vi "Enable_AFR_EGT_Graph (SubVI).vi"(0 "Leistungsgraph":refnum<vi>, 1 "AFR EGT":bool, 2 "Y-Koord. Graph-Reset-Button (782)":i32, 3 "Lambda":refnum<vi>, 5 "Reset Skalierung":refnum<vi>, 7 "Höhe Leistungs-Graph (646)":u32, 9 "AFR EGT Gaph":refnum<vi>, 12 "AFR":refnum<vi>, 13 "EGT [°C]":refnum<vi>, 14 "Skalierungsfaktor Leistungsgraph":dbl) -> ()   [LabVIEW 2014]
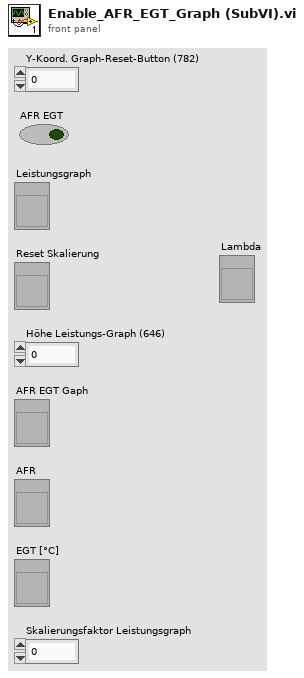
[diagram p1: front panel]
types:
  T1 = typedef "LVRangeTypeDef.ctl" = cluster{"Minimum":dbl, "Maximum":dbl, "Increment":dbl, "Minor Increment":dbl, "Start":dbl}
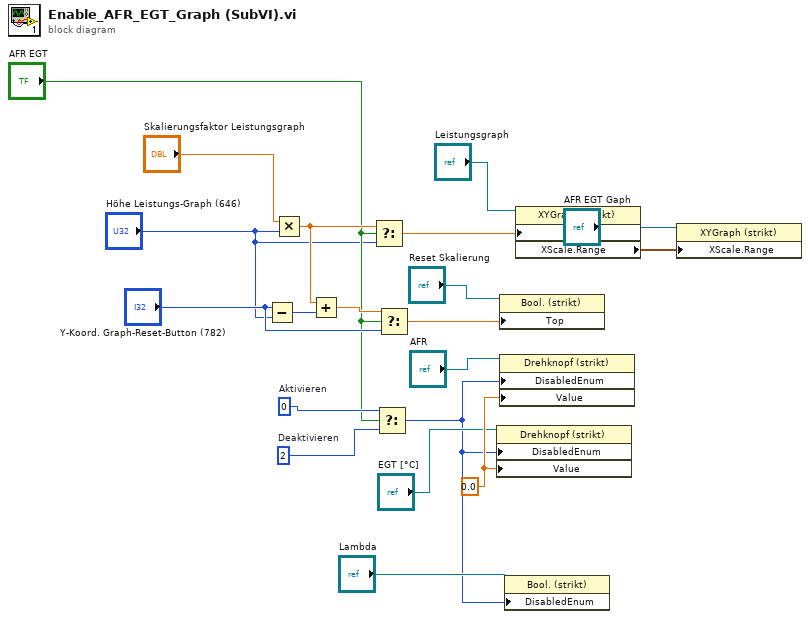
[diagram p0: block diagram]
diagram:
  w20 = 0  # Aktivieren
  w9 = 0.0
  w15 = 2  # Deaktivieren
  n1 = Subtract(x="Y-Koord. Graph-Reset-Button (782)", y="Höhe Leistungs-Graph (646)") -> (x-y=w16:u32)
  n2 = Multiply(x="Skalierungsfaktor Leistungsgraph", y="Höhe Leistungs-Graph (646)") -> (x*y=w17:dbl)
  n3 = Add(x=w17, y=w16) -> (x+y=w18:dbl)
  n4 = Select(t=w17, s="AFR EGT", f="Höhe Leistungs-Graph (646)") -> (s? t:f=w11:dbl)
  n5 = Select(t=w20, s="AFR EGT", f=w15) -> (s? t:f=w1:i32)
  n6 = Select(t=w18, s="AFR EGT", f="Y-Koord. Graph-Reset-Button (782)") -> (s? t:f=w14:dbl)
  n7 = property on="Eigenschaftsknoten" class="Drehknopf (strikt)"(reference="EGT [°C]", "DisabledEnum"=w1, "Value"=w9) -> ()  [unwired: 1 in, 2 out]
  n8 = property on="Eigenschaftsknoten" class="Bool. (strikt)"(reference="Reset Skalierung", "Top"=w14) -> ()  [unwired: 1 in, 2 out]
  n9 = property on="Eigenschaftsknoten" class="Drehknopf (strikt)"(reference="AFR", "DisabledEnum"=w1, "Value"=w9) -> ()  [unwired: 1 in, 2 out]
  n10 = property on="Eigenschaftsknoten" class="Bool. (strikt)"(reference="Lambda", "DisabledEnum"=w1) -> ()  [unwired: 1 in, 2 out]
  n11 = property on="Eigenschaftsknoten" class="XYGraph (strikt)"(reference="Leistungsgraph", "Height"=w11) -> ("XScale.Range"=w8:T1)  [unwired: 1 in, 2 out]
  n12 = property on="Eigenschaftsknoten" class="XYGraph (strikt)"(reference="AFR EGT Gaph", "XScale.Range"=w8) -> ()  [unwired: 1 in, 2 out]
